vi "Osc_DMM_Initilize.vi"(4 "Scan Measure\nTime":dbl=2e-05, 6 "Measure Maximun Voltage":dbl=100.0 format="%#_13g", 8 "error in (no error)":errorcluster, 9 "Trigger Count (1)":i32=1 format="%#.6g", 10 "Sample Count (1)":i32=1 format="%#.6g", 11 "VISA Refnum in":refnum<visa-resource-name>) -> (0 "error out":errorcluster, 3 "VISA Refnum out":refnum<visa-resource-name>)   [LabVIEW 2023]
uses:
  <instrlib>/Agilent 3446X Series/Agilent 3446X Series.lvlib
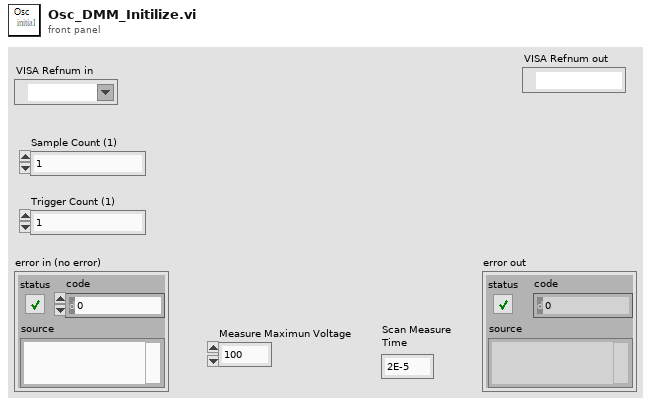
[diagram p1: front panel]
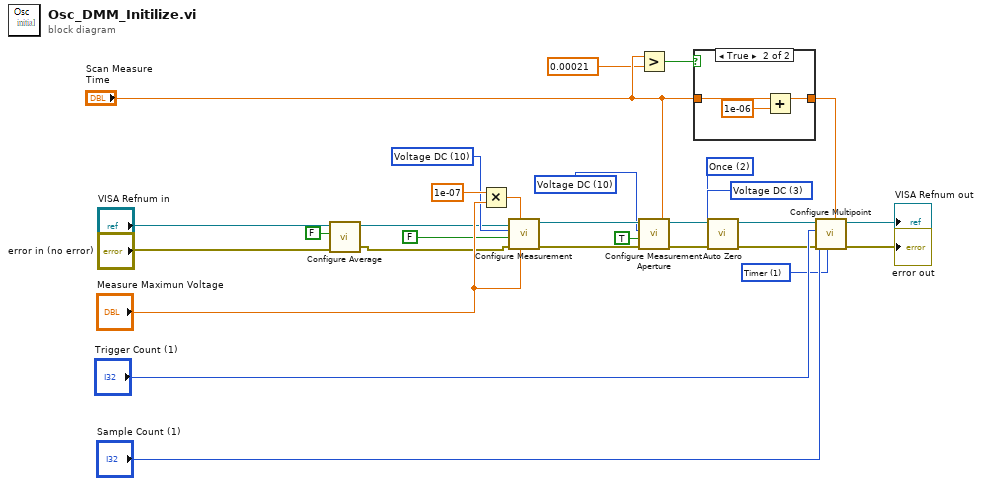
[diagram p0: block diagram]
diagram:
  w13 = 1 items=["Immediate", "Timer"] ("Sample Source (0: Immediate)")
  w15 = 10 items=["Continuity", "Current AC", "Current DC", "Diode", "Frequency", "Resistance 4-wire", "Period", "Resistance 2-wire", "Temperature", "Voltage AC", "Voltage DC", "Voltage DC Ratio", "Capacitance"] ("Measurement Function (10: Voltage DC)")
  w24 = 3 items=["Current DC", "Resistance", "Temperature", "Voltage DC"] ("Zero Type (0: Current DC)")
  w23 = 2 items=["Disable", "Enable", "Once"] ("Auto Zero (1: Enable)")
  w21 = 10 items=["Continuity", "Current AC", "Current DC", "Diode", "Frequency", "Resistance 4-wire", "Period", "Resistance 2-wire", "Temperature", "Voltage AC", "Voltage DC", "Voltage DC Ratio", "Capacitance"] ("Measurement Function (0: Continuity)")
  n1 = call <instrlib>:"Configure Average.vi"("error in (no error)"="error in (no error)", "Enable Statistics (F: Disable)"=FALSE, "VISA resource name"="VISA Refnum in") -> ("error out"=w11:errorcluster, "VISA resource name out"=w12:refnum<visa-resource-name>)  [unwired: 7 in]
  n2 = Multiply(x=1e-07, y="Measure Maximun Voltage") -> (x*y=w16:dbl)
  n3 = call <instrlib>:"Configure Measurement.vi"("Manual Range (1)"="Measure Maximun Voltage", "Absolute Resolution (1E-6)"=w16, "error in (no error)"=w11, "Auto Range (T: Enable)"=FALSE, "Measurement Function (10: Voltage DC)"=w15, "VISA resource name"=w12) -> ("error out"=w29:errorcluster, "VISA resource name out"=w28:refnum<visa-resource-name>)  [unwired: 4 out]
  n4 = Greater?(x="Scan Measure\nTime", y=0.00021) -> (0:w3:bool)
  n5 = call <instrlib>:"Configure Measurement Aperture.vi"("Aperture Time (0.1s)"="Scan Measure\nTime", "error in (no error)"=w29, "Enable Aperture (F: Disable)"=TRUE, "Measurement Function (0: Continuity)"=w21, "VISA resource name"=w28) -> ("error out"=w25:errorcluster, "VISA resource name out"=w27:refnum<visa-resource-name>)  [unwired: 5 in]
  n6 = case shown="True" w3 {
    tunnel: "Scan Measure\nTime" -> [w30 w33]
    tunnel: [w30 w32] -> w4
    frame False {
    }
    frame True {
      n7 = Add(x=w33, y=1e-06) -> (x+y=w32:dbl)
    }
  }
  n8 = call <instrlib>:"Auto Zero.vi"("error in (no error)"=w25, "Auto Zero (1: Enable)"=w23, "Zero Type (0: Current DC)"=w24, "VISA resource name"=w27) -> ("error out"=w9:errorcluster, "VISA resource name out"=w10:refnum<visa-resource-name>)  [unwired: 6 in]
  n9 = call <instrlib>:"Configure Multipoint.vi"("Sample Interval (1 Second)"=w4, "Sample Source (0: Immediate)"=w13, "error in (no error)"=w9, "Sample Count (1)"="Sample Count (1)", "Trigger Count (1)"="Trigger Count (1)", "VISA resource name"=w10) -> ("error out"=→"error out":errorcluster, "VISA resource name out"=→"VISA Refnum out":refnum<visa-resource-name>)  [unwired: 1 in, 3 out]
